vi "AddTestToMap.vi"(8 "error in (no error)":errorcluster, 9 "Test":refnum<class "Test.lvclass">, 10 "Tag":string, 11 "ResultTreeListener in":refnum<class "ResultTreeListener.lvclass">) -> (0 "error out":errorcluster, 3 "ResultTreeListener out":refnum<class "ResultTreeListener.lvclass">)   [LabVIEW 2017, in "ResultTreeListener.lvclass"]
doc: "Adds a test to the test map."
uses:
  ResultTreeListener.lvclass
  Test/Test.lvclass
  ResultTreeListener.lvclass/ResultTreeListener.ctl
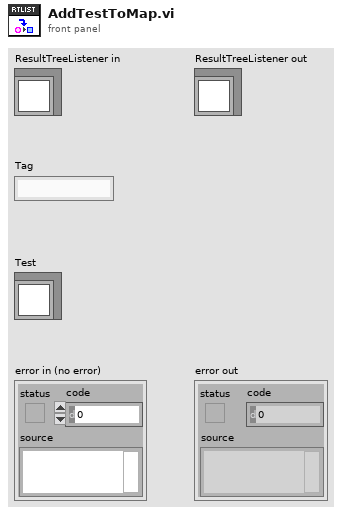
[diagram p1: front panel]
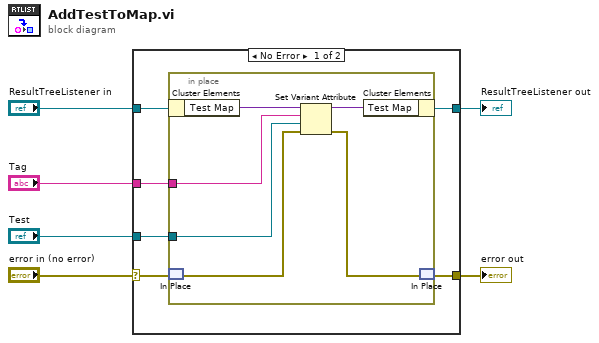
[diagram p0: block diagram]
diagram:
  n1 = case shown="No Error" "error in (no error)" {
    selector: "error in (no error)" -> [w8 w20]
    tunnel: [w7 w20] -> w5
    tunnel: [w11 w19] -> w3
    tunnel: "ResultTreeListener in" -> [w12 w19]
    tunnel: "Tag" -> [w10 _]
    tunnel: "Test" -> [w9 _]
    frame No Error {
      n2 = in-place {
        in-place-border: w10 -> [w16]
        in-place-border: w9 -> [w15]
        n3 = in-place-cluster #1(w12) -> ("Test Map"=w18:variant)
        n4 = in-place-match #2(w8) -> (w14:errorcluster)
        n5 = Set Variant Attribute(Variant=w18, name=w16, value=w15, error in=w14) -> (Variant out=w17:variant, error out=w13:errorcluster)  [unwired: 1 out]
        n6 = in-place-cluster #1("Test Map"=w17) -> (w11:refnum<class "ResultTreeListener.lvclass">)
        n7 = in-place-match #2(w13) -> (w7:errorcluster)
      }
    }
    frame Error {
    }
  }
  "error out" <- w5
  "ResultTreeListener out" <- w3
